vi "1-pickup.vi"() -> ()   [LabVIEW 2015]
uses:
  <vilib>/myRIO/Instrument Drivers/Onboard IO/DIO/typedefs/DIO Reference.ctl
  <vilib>/myRIO/Common/Instrument Driver Framework/Utilities/typedefs/myRIO Generic Hardware Reference.ctl
  <vilib>/myRIO/Common/Instrument Driver Framework/Utilities/typedefs/Hardware Version Enum.ctl
  <vilib>/myRIO/Common/Instrument Driver Framework/Utilities/typedefs/myRIO v1.0 Reference.ctl
  <vilib>/myRIO/Common/Instrument Driver Framework/Utilities/typedefs/Generic FPGA Reference.ctl
  <vilib>/myRIO/Common/Instrument Driver Framework/myRIO v1.0/DIO/typedefs/DIO Channels List.ctl
  <vilib>/myRIO/Common/Instrument Driver Framework/myRIO v1.0/DIO/typedefs/DIO Channels Enum.ctl
  <vilib>/userdefined/High Color/nirio_resource_hc.ctl
  <vilib>/myRIO/Instrument Drivers/Onboard IO/PWM/typedefs/PWM Reference.ctl
  <vilib>/myRIO/Common/Instrument Driver Framework/myRIO v1.0/PWM/typedefs/PWM Channels Enum.ctl
  <vilib>/myRIO/Instrument Drivers/Onboard IO/PWM/typedefs/PWM Configuration.ctl
  <vilib>/myRIO/Common/Instrument Driver Framework/Utilities/vis/Is FPGA Ref Available.vi
  <vilib>/myRIO/Common/Instrument Driver Framework/myRIO v1.0/PWM/vis/myRIO v1.1 Open PWM.vi
  <vilib>/myRIO/Instrument Drivers/Onboard IO/PWM/vis/Set Duty Cycle and Frequency.vi
  <vilib>/myRIO/Common/Instrument Driver Framework/myRIO v1.0/DIO/vis/myRIO v1.1 Open DIO.vi
  <vilib>/myRIO/Instrument Drivers/Onboard IO/DIO/vis/Write.vi
  <vilib>/myRIO/Instrument Drivers/Onboard IO/DIO/vis/Read.vi
  <vilib>/myRIO/Common/Instrument Driver Framework/Utilities/vis/Validate Channels.vi
  <vilib>/myRIO/Common/Instrument Driver Framework/myRIO v1.0/PWM/vis/myRIO v1.0 Reserve PWM.vi
  <vilib>/myRIO/Common/Instrument Driver Framework/myRIO v1.0/DIO/vis/myRIO v1.0 Reserve DIO.vi
  <vilib>/myRIO/Common/Instrument Driver Framework/myRIO v1.0/PWM/vis/myRIO v1.0 Build MUX Configuration PWM.vi
  <vilib>/myRIO/Common/Instrument Driver Framework/myRIO v1.0/Resource Manager/vis/myRIO v1.0 Reserve Channel List.vi
  <vilib>/myRIO/Common/Instrument Driver Framework/myRIO v1.0/DIO/vis/myRIO v1.0 Build MUX Configuration DIO.vi
  <vilib>/myRIO/Common/Instrument Driver Framework/myRIO v1.0/Resource Manager/vis/myRIO v1.0 Create Configuration List.vi
  <vilib>/myRIO/Common/Instrument Driver Framework/myRIO v1.0/Resource Manager/vis/myRIO v1.0 Reserve Channel.vi
  <vilib>/myRIO/Common/Instrument Driver Framework/myRIO v1.0/Resource Manager/vis/myRIO v1.0 Unreserve Channel.vi
  <vilib>/myRIO/Common/Instrument Driver Framework/myRIO v1.0/Resource Manager/vis/myRIO v1.0 Build Mutex Name.vi
  <vilib>/Utility/VariantDataType/GetNumericInfo.vi
  <vilib>/Utility/error.llb/Error Cluster From Error Code.vi
  <vilib>/myRIO/Common/Instrument Driver Framework/myRIO v1.0/myRIO v1.1 Open.vi
  <vilib>/myRIO/Common/Instrument Driver Framework/Utilities/vis/IO Manager.vi
  <vilib>/myRIO/Common/Instrument Driver Framework/Utilities/vis/Configuration Manager.vi
  <vilib>/myRIO/Common/Instrument Driver Framework/myRIO v1.0/Resource Manager/vis/myRIO v1.0 Configure IO.vi
  <vilib>/myRIO/Common/Instrument Driver Framework/myRIO v1.0/myRIO v1.0 Close.vi
  <vilib>/myRIO/Common/Instrument Driver Framework/myRIO v1.0/DIO/vis/myRIO v1.0 Read DIO.vi
  <vilib>/myRIO/Common/Instrument Driver Framework/myRIO v1.0/DIO/vis/myRIO v1.0 Write DIO.vi
  <vilib>/myRIO/Common/Instrument Driver Framework/myRIO v1.0/PWM/vis/myRIO v1.0 Write PWM.vi
  <vilib>/myRIO/Express VI/Onboard IO/DI/DI Express VI.xnode
  <vilib>/myRIO/Instrument Drivers/Onboard IO/DIO/vis/myRIO DIO Open.xnode
  <vilib>/myRIO/Express VI/Onboard IO/DO/DO Express VI.xnode
  <vilib>/myRIO/Express VI/Onboard IO/PWM/PWM Express VI.xnode
  <vilib>/myRIO/Instrument Drivers/Onboard IO/PWM/vis/myRIO PWM Open.xnode
  <vilib>/myRIO/Instrument Drivers/Onboard IO/DIO/DIO.lvlib
  <vilib>/myRIO/Instrument Drivers/Onboard IO/PWM/PWM.lvlib
  class/Car.lvclass
  class/SonarSensor.lvclass
panel:
  out "Distance":dbl
  out "Time of Flight Front":u32
  in  "stop":bool
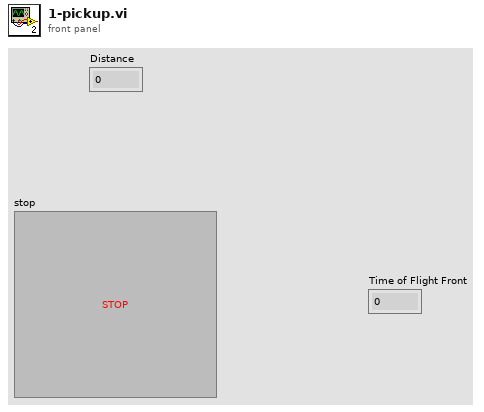
[diagram p1: front panel]
types:
  T1 = typedef "PWM.lvlib/PWM Reference.ctl" = cluster{"myRIO Reference":T2, "PWM Channels Enum":T6, "PWM Configuration":T7}
  T2 = typedef "myRIO Generic Hardware Reference.ctl" = cluster{"myRIO Model":T3, "myRIO Hardware Reference":T4}
  T3 = typedef "Hardware Version Enum.ctl" = enum16{"Unknown", "myRIO-1900", "myRIO-1950", "roboRIO"}
  T4 = typedef "myRIO v1.0 Reference.ctl" = cluster{"Generic FPGA Reference":T5, "Allow multiple opens":bool}
  T5 = typedef "Generic FPGA Reference.ctl" = refnum<k20>
  T6 = typedef "PWM Channels Enum.ctl" = enum16{"Not Connected", "C/PWM0", "C/PWM1", "A/PWM0", "A/PWM1", "A/PWM2", "B/PWM0", "B/PWM1", "B/PWM2", "PWM/PWM0", "PWM/PWM1", "PWM/PWM2", "PWM/PWM3", "PWM/PWM4", "PWM/PWM5", "PWM/PWM6", "PWM/PWM7", "PWM/PWM8", "PWM/PWM9"}
  T7 = typedef "PWM.lvlib/PWM Configuration.ctl" = cluster{"Frequency":dbl, "Duty Cycle":dbl}
  T8 = typedef "nirio_resource_hc.ctl" = tag
  T9 = typedef "DIO.lvlib/DIO Reference.ctl" = cluster{"myRIO Reference":T2, "DIO Channels List":T10}
  T10 = typedef "DIO Channels List.ctl" = T11[]
  T11 = typedef "DIO Channels Enum.ctl" = enum16{"Not Connected", "C/DIO0", "C/DIO1", "C/DIO2", "C/DIO3", "C/DIO4", "C/DIO5", "C/DIO6", "C/DIO7", "A/DIO0", "A/DIO1", "A/DIO2", "A/DIO3", "A/DIO4", "A/DIO5", "A/DIO6", "A/DIO7", "A/DIO8", "A/DIO9", "A/DIO10", "A/DIO11", "A/DIO12", "A/DIO13", "A/DIO14", "A/DIO15", "B/DIO0", "B/DIO1", "B/DIO2", "B/DIO3", "B/DIO4", "B/DIO5", "B/DIO6", "B/DIO7", "B/DIO8", "B/DIO9", "B/DIO10", "B/DIO11", "B/DIO12", "B/DIO13", "B/DIO14", "B/DIO15", "LED0", "LED1", "LED2", "LED3", "Button0", "DIO/DIO0", "DIO/DIO1", "DIO/DIO2", "DIO/DIO3", "DIO/DIO4", "DIO/DIO5", "DIO/DIO6", "DIO/DIO7", "DIO/DIO8", "DIO/DIO9", "SPI/CS0", "SPI/CS1", "SPI/CS2", "SPI/CS3", "LED RADIO (Green)", "LED RADIO (Red)", "LED COMM (Green)", "LED COMM (Red)", "LED MODE (Green)", "LED MODE (Red)"}
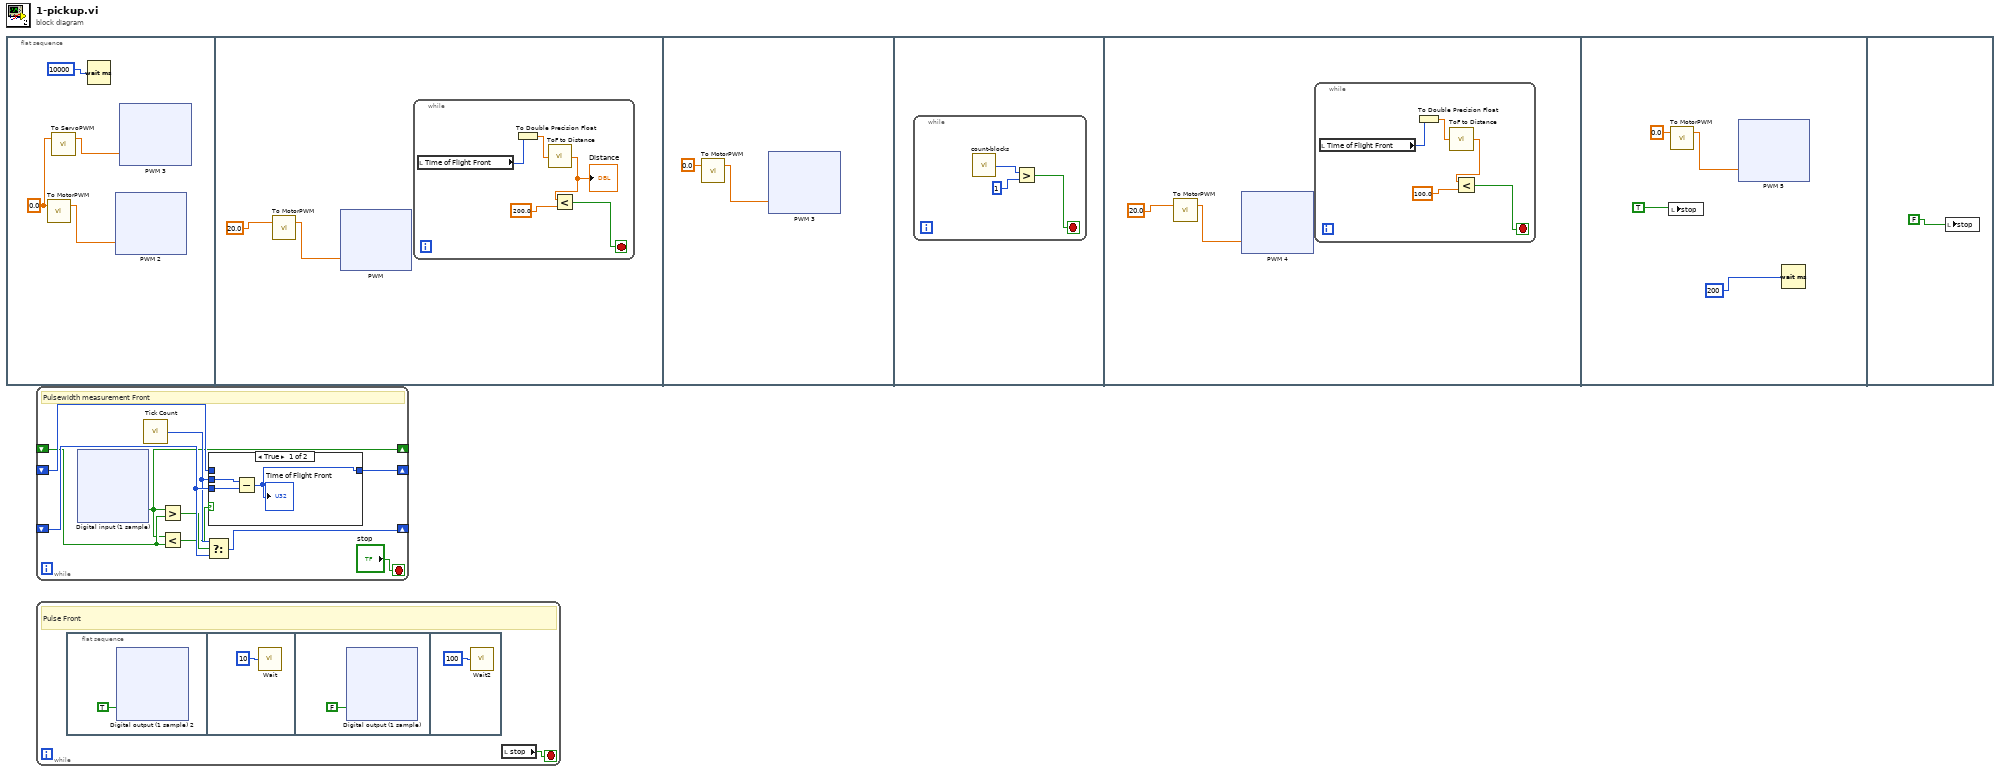
[diagram p0: block diagram]
diagram:
  n1 = flat-sequence {
    frame #0 {
      w3 = 0.0 ("Speed")
      n2 = call "To MotorPWM.vi"("Speed"=w3) -> ("MotorPWM"=w4:dbl)  [unwired: 1 in, 1 out]
      n3 = call "To ServoPWM.vi"("Wheel Angle"=w3) -> ("ServoPWM"=w2:dbl)  [unwired: 1 in, 1 out]
      n4 = Wait (ms)(milliseconds to wait=10000) -> ()  [unwired: 1 out]
      n5 = xnode "PWM 2"("Duty Cycle"=w4) -> ()  [unwired: 1 in, 1 out]
      n6 = xnode "PWM 3"("Duty Cycle"=w2) -> ()  [unwired: 1 in, 1 out]
    }
    frame #1 {
      n7 = call "To MotorPWM.vi"("Speed"=20.0) -> ("MotorPWM"=w76:dbl)  [unwired: 1 in, 1 out]
      n8 = xnode "PWM"("Duty Cycle"=w76) -> ()  [unwired: 1 in, 1 out]
      n9 = while {
        stop <- w77 stop-if-true
        n10 = local read "Time of Flight Front"() -> (w81:u32)
        n11 = To Double Precision Float(number=w81) -> (double precision float=w80:dbl)
        n12 = call "ToF to Distance.vi"("Time of Flight"=w80) -> ("Distance"=w79:dbl)
        "Distance" <- w79
        n13 = Less?(x=w79, y=200.0) -> (x < y?=w77:bool)
      }
    }
    frame #2 {
      n14 = call "To MotorPWM.vi"("Speed"=0.0) -> ("MotorPWM"=w118:dbl)  [unwired: 1 in, 1 out]
      n15 = xnode "PWM 3"("Duty Cycle"=w118) -> ()  [unwired: 1 in, 1 out]
    }
    frame #3 {
      n16 = while {
        stop <- w154 stop-if-true
        n17 = call "count-blocks.vi"() -> ("block count"=w156:i32)
        n18 = Greater?(x=w156, y=1) -> (0:w154:bool)
      }
    }
    frame #4 {
      n19 = call "To MotorPWM.vi"("Speed"=20.0) -> ("MotorPWM"=w158:dbl)  [unwired: 1 in, 1 out]
      n20 = xnode "PWM 4"("Duty Cycle"=w158) -> ()  [unwired: 1 in, 1 out]
      n21 = while {
        stop <- w159 stop-if-true
        n22 = local read "Time of Flight Front"() -> (w163:u32)
        n23 = To Double Precision Float(number=w163) -> (double precision float=w162:dbl)
        n24 = call "ToF to Distance.vi"("Time of Flight"=w162) -> ("Distance"=w161:dbl)
        n25 = Less?(x=w161, y=100.0) -> (x < y?=w159:bool)
      }
    }
    frame #5 {
      n26 = local write "stop"(TRUE) -> ()
      n27 = call "To MotorPWM.vi"("Speed"=0.0) -> ("MotorPWM"=w202:dbl)  [unwired: 1 in, 1 out]
      n28 = xnode "PWM 5"("Duty Cycle"=w202) -> ()  [unwired: 1 in, 1 out]
      n29 = Wait (ms)(milliseconds to wait=200) -> ()  [unwired: 1 out]
    }
    frame #6 {
      n30 = local write "stop"(FALSE) -> ()
    }
  }
  n31 = while "Pulsewidth Measurement + Sound Output" {
    shift-left: _ -> [w248]
    shift-right: [w241] -> _
    shift-left: _ -> [w247]
    shift-right: [w246] -> _
    shift-left: _ -> [w244]
    shift-right: [w239] -> _
    stop <- "stop" stop-if-true
    # "Pulsewidth measurement Front"
    n32 = xnode "Digital input (1 sample)"() -> ("B/DIO7 (Pin 25)"=w239:bool)  [unwired: 1 in, 1 out]
    n33 = call "Tick Count"() -> ("Tick Count(uSec)"=w243:u32)
    n34 = Greater?(x=w239, y=w244) -> (0:w245:bool)
    n35 = Less?(x=w239, y=w244) -> (x < y?=w242:bool)
    n36 = Select(t=w243, s=w245, f=w247) -> (s? t:f=w246:u32)
    n37 = case shown="True" w242 {
      tunnel: w248 -> [_ w287]
      tunnel: w243 -> [w285 _]
      tunnel: w247 -> [w286 _]
      tunnel: [w284 w287] -> w241
      frame True {
        n38 = Subtract(x=w285, y=w286) -> (x-y=w284:u32)
        "Time of Flight Front" <- w284
      }
      frame False {
      }
    }
  }
  n39 = while {
    stop <- w288 stop-if-true
    # "Pulse Front"
    n40 = flat-sequence {
      frame #0 {
        n41 = xnode "Digital output (1 sample) 2"("B/DIO4 (Pin 19)"=TRUE ("ConnectorB/DIO4")) -> ()  [unwired: 1 in, 1 out]
      }
      frame #1 {
        n42 = call "Wait"("Count(uSec)"=u32 10 ("Count(mSec)")) -> ()  [unwired: 1 out]
      }
      frame #2 {
        n43 = xnode "Digital output (1 sample)"("B/DIO4 (Pin 19)"=FALSE ("ConnectorB/DIO4")) -> ()  [unwired: 1 in, 1 out]
      }
      frame #3 {
        n44 = call "Wait2"("Count(mSec)"=u32 100) -> ()  [unwired: 1 out]
      }
    }
    n45 = local read "stop"() -> (w288:bool)
  }
